vi "Drive Turn.vi"(4 "Angle":dbl, 5 "Left Input":dbl, 7 "Right Input":dbl) -> (0 "Left Output":dbl, 1 "Right Output":dbl)   [LabVIEW 2013]
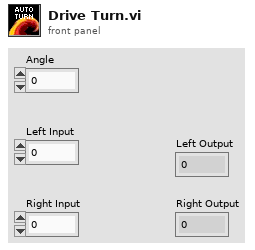
[diagram p1: front panel]
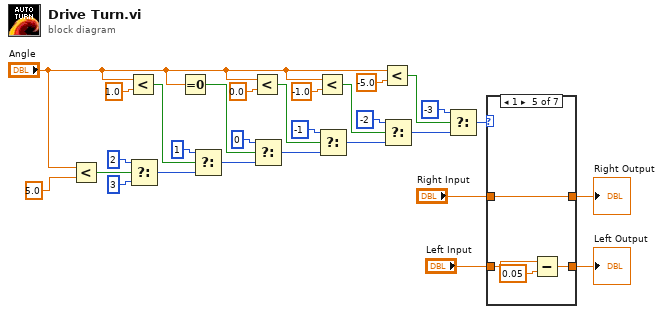
[diagram p0: block diagram]
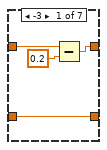
[diagram p2: hidden frame]
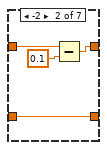
[diagram p3: hidden frame]
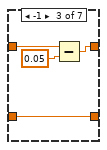
[diagram p4: hidden frame]
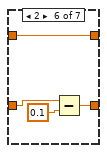
[diagram p6: hidden frame]
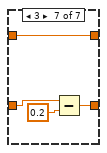
[diagram p7: hidden frame]
diagram:
  n1 = Less?(x="Angle", y=5.0) -> (x < y?=w23:bool)
  n2 = Less?(x="Angle", y=1.0) -> (x < y?=w21:bool)
  n3 = Select(t=i8 2, s=w23, f=i8 3) -> (s? t:f=w15:i8)
  n4 = Equal To 0?(x="Angle") -> (x = 0?=w11:bool)
  n5 = Select(t=i8 1, s=w21, f=w15) -> (s? t:f=w9:i8)
  n6 = Less?(x="Angle", y=0.0) -> (x < y?=w24:bool)
  n7 = Select(t=i8 0, s=w11, f=w9) -> (s? t:f=w8:i8)
  n8 = Less?(x="Angle", y=-1.0) -> (x < y?=w26:bool)
  n9 = Select(t=i8 -1, s=w24, f=w8) -> (s? t:f=w19:i8)
  n10 = Less?(x="Angle", y=-5.0) -> (x < y?=w28:bool)
  n11 = Select(t=i8 -2, s=w26, f=w19) -> (s? t:f=w20:i8)
  n12 = Select(t=i8 -3, s=w28, f=w20) -> (s? t:f=w7:i8)
  n13 = case shown="1" w7 {
    tunnel: "Right Input" -> [w33 w36 w40 w43 w46 w48 w52]
    tunnel: [w31 w35 w39 w43 w46 w48 w52] -> w4
    tunnel: "Left Input" -> [w30 w37 w41 w42 w45 w51 w55]
    tunnel: [w30 w37 w41 w42 w44 w49 w53] -> w2
    frame -3 {
      n14 = Subtract(x=w33, y=0.2) -> (x-y=w31:dbl)
    }
    frame -2 {
      n15 = Subtract(x=w36, y=0.1) -> (x-y=w35:dbl)
    }
    frame -1 {
      n16 = Subtract(x=w40, y=0.05) -> (x-y=w39:dbl)
    }
    frame 0, Default {
    }
    frame 1 {
      n17 = Subtract(x=w45, y=0.05) -> (x-y=w44:dbl)
    }
    frame 2 {
      n18 = Subtract(x=w51, y=0.1) -> (x-y=w49:dbl)
    }
    frame 3 {
      n19 = Subtract(x=w55, y=0.2) -> (x-y=w53:dbl)
    }
  }
  "Left Output" <- w2
  "Right Output" <- w4
